vi "ADO Connection Get Properties.vi"(8 "error in (no error)":errorcluster caption="错误输入（无错误）", 11 "Database Connection 输入":refnum<class "Database Connection.lvclass"> caption="DNL_LabVIEW Object in") -> (0 "error out":errorcluster caption="错误输出", 1 "connection properties":T1, 3 "Database Connection 输出":refnum<class "Database Connection.lvclass"> caption="DNL_LabVIEW Object out")   [LabVIEW 2011, in "Database Connection.lvclass"]
uses:
  Database Connection.lvclass
  Database Connection.lvclass/Database Connection.ctl
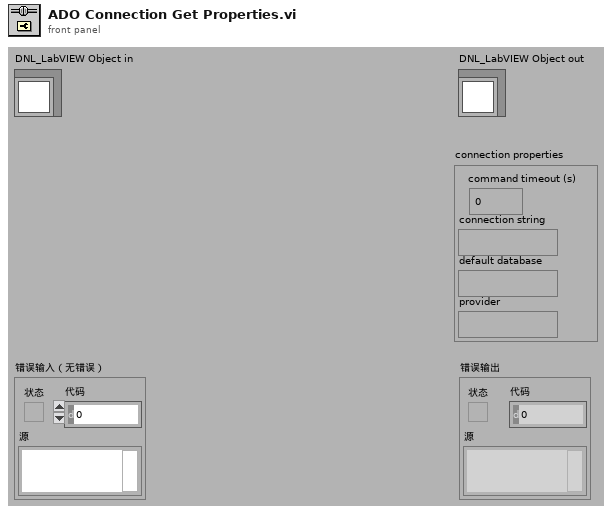
[diagram p1: front panel]
types:
  T1 = cluster{"command timeout (s)":i32, "connection string":string, "default database":string, "provider":string}
  T2 = cluster{"CommandTimeout":i32, "ConnectionString":string, "DefaultDatabase":string, "Provider":string}
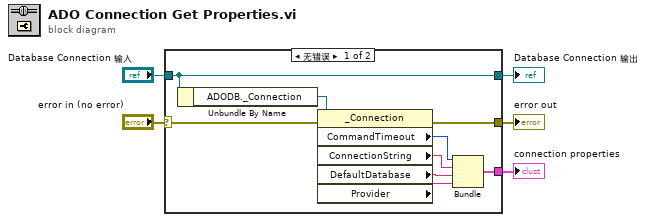
[diagram p0: block diagram]
diagram:
  n1 = case shown="无错误" "error in (no error)" {
    selector: "error in (no error)" -> [w7 w16]
    tunnel: [w6 w16] -> w4
    tunnel: [w14 w15] -> w2
    tunnel: "Database Connection 输入" -> [w14 w15]
    tunnel: [w8 _] -> w1
    frame No Error {
      n2 = Unbundle By Name(w14) -> ("ADODB._Connection"=w13:refnum<k7>)
      n3 = property class="_Connection"(reference=w13, error in=w7) -> (error out=w6:errorcluster, "CommandTimeout"=w12:i32, "ConnectionString"=w11:string, "DefaultDatabase"=w10:string, "Provider"=w9:string)  [unwired: 1 out]
      n4 = Bundle("CommandTimeout"=w12, "ConnectionString"=w11, "DefaultDatabase"=w10, "Provider"=w9) -> (w8:T2)  [unwired: 1 in]
    }
    frame Error {
    }
  }
  "error out" <- w4
  "Database Connection 输出" <- w2
  "connection properties" <- w1
